vi "KMCS2000 Create graph.vi"(9 "Array":ext[][](array[numeric]), 10 "y index":i32, 11 "x index":i32) -> (3 "XY Graph":cluster{"X":dbl[], "Y":dbl[]}[](array[cluster]))   [LabVIEW 2018]
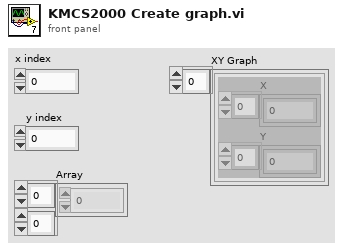
[diagram p1: front panel]
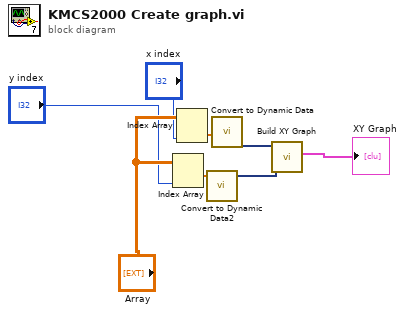
[diagram p0: block diagram]
diagram:
  n1 = Index Array(array="Array", index (col)="y index") -> (element=w6:ext[])  [unwired: 1 in]
  n2 = Index Array(array="Array", index (col)="x index") -> (element=w4:ext[])  [unwired: 1 in]
  n3 = call "Convert to Dynamic Data2"("Array"=w6) -> ("Dynamic Data Type"=w7:dynamicdata)  [unwired: 3 in]
  n4 = call "Convert to Dynamic Data"("Array"=w4) -> ("Dynamic Data Type"=w3:dynamicdata)  [unwired: 3 in]
  n5 = call "Build XY Graph"("Y Input"=w7, "X Input"=w3) -> ("XY Graph"=→"XY Graph":cluster{"X":dbl[], "Y":dbl[]}[])  [unwired: 8 in, 1 out]
